vi "Get Pressure.vi"() -> ()   [LabVIEW 2017]
uses:
  Robot Global Data.vi
panel:
  out "Pressure":dbl
  out "Presure Voltage":dbl
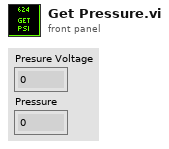
[diagram p1: front panel]
types:
  T1 = typedef "Dashboard Control Data.ctl" = cluster{"Drivetrain Settings Cluster":T2, "Intake Presets":T4, "Elevator Settings Cluster":T5, "Drivetrain Encoder Values":T7, "Auton Chooser":T8, "Auton Presets":cluster{"Start Position":dbl}, "Elevator Encoder Values":T9, "Pressure M":dbl, "Pressure B":dbl}
  T2 = typedef "Drivetrain Settings Cluster.ctl" = cluster{"Gyro Steer PID Gains":T3, "Distance Drive PID Gains":T3, "Drive Tolerance":dbl, "Gyro Tolerance":dbl, "Gyro Output":dbl, "Distance Output":dbl, "Y Power Multiplier":dbl, "Turn Power Multiplier":dbl, "Creep Rate":dbl, "Encoder Reset":bool, "DT Mode Modifier":enum16{"None, Default", "Cube", "Square"}, "Left Encoder Tick Constant":dbl, "Right Encoder Tick Constant":dbl, "Shift Speed":dbl, "Zero Gyro":bool}
  T3 = typedef "PID Gains Cluster.ctl" = cluster{"Integral Time":dbl, "Proportional Gain":dbl, "Derivative Time":dbl}
  T4 = typedef "Intake Presets.ctl" = cluster{"Idle Angle":dbl, "Mid Angle":dbl, "Low Angle":dbl, "Outtake Power":dbl, "Intake Power":dbl, "Unstuck":dbl, "Angle Tolerance":dbl, "Max Angle":dbl, "Max Current":dbl, "Current Trip Time":dbl, "Reset Encoder?":bool, "Encoder Scale":dbl, "PID gains":cluster{"proportional gain (Kc)":dbl, "integral time (Ti, min)":dbl, "derivative time (Td, min)":dbl}, "output range":cluster{"output high":dbl, "output low":dbl}, "IR Constant Pull Rate":dbl}
  T5 = typedef "Elevator Settings Cluster.ctl" = cluster{"Ground Height":dbl, "Switch Height":dbl, "Scale High Height ":dbl, "Scale Low Height":dbl, "Elevator PID Gains":T6, "Elevator Tolerance":dbl, "Reset Encoders":bool, "Encoder Scale":dbl, "Max Height":dbl, "Mid Height":dbl, "output range":cluster{"output high":dbl, "output low":dbl}, "Slow Down Tolerance":dbl, "Tick Constant":dbl, "Anti-tip Multiplier":dbl, "Slow Down Multiplier":dbl}
  T6 = typedef "PID Gains.ctl" = cluster{"proportional gain (Kc)":dbl, "integral time (Ti, min)":dbl, "derivative time (Td, min)":dbl}
  T7 = typedef "DT Encoder Values.ctl" = cluster{"Left Encoder":cluster{"Distance":dbl, "Speed":dbl, "Tick":dbl}, "Right Encoder":cluster{"Distance":dbl, "Speed":dbl, "Tick":dbl}}
  T8 = typedef "Auton Chooser.ctl" = cluster{"Left":bool, "Center":bool, "Right":bool, "Scale":bool, "Both":bool, "Switch":bool}
  T9 = typedef "Elevator Encoder Values.ctl" = cluster{"Encoder Values":cluster{"Distance":dbl, "Speed":dbl, "Tick":dbl}}
  T10 = typedef "WPI_AnalogChannelDevRef.ctl" = cluster{"DevStatus":errorcluster, "Analog Channel":T11}
  T11 = typedef "FPGA_AIChannel.ctl" = enum8{"AI 0", "AI 1", "AI 2", "AI 3", "AI MXP 0", "AI MXP 1", "AI MXP 2", "AI MXP 3", "Invalid"}
  T12 = typedef "Dashboard Status Data.ctl" = cluster{"Elevator Status Cluster":T13, "Drivetrain Status Cluster":T16, "Intake Status Cluster":T18, "Climb Status Cluster":T21, "Intake PDP Info":T22, "Auton Command Cluster":T23, "Pressure ":dbl}
  T13 = typedef "Elevator Status Cluster.ctl" = cluster{"Finished":bool, "Elevator Power":dbl, "Elevator State":T14, "Elevator Mode":T15, "Elevator Height":dbl, "At Bottom?":bool, "At Top?":bool, "Scale high?":bool, "PID Output":dbl}
  T14 = typedef "Elevator State.ctl" = enum16{"Idle", "Ground", "Mid", "Scale", "Switch"}
  T15 = typedef "Elevator Mode.ctl" = enum16{"Semi Auto", "Manual", "Auto"}
  T16 = typedef "Drivetrain Status Cluster.ctl" = cluster{"Throttle (Y)":dbl, "Steer (X)":dbl, "Drivetrain Mode":T17, "Brake?":bool, "Distance Drive Complete?":bool, "PID Drive Complete?":bool, "Creep Mode?":bool, "Gyro Steer Complete?":bool, "Gyro":dbl, "X Max Output":dbl, "X Min Output":dbl, "Y Max Output ":dbl, "Y Min Output":dbl, "Heading Target":dbl, "Distance Target":dbl, "2nd Gear":bool, "Drivetrain Encoder Values":T7}
  T17 = typedef "Drivetrain Mode.ctl" = enum16{"Manual", "Gyro Steer", "PID Drive", "Distance Drive", "Autonomous"}
  T18 = typedef "Intake Status Cluster.ctl" = cluster{"Intake Mode":T19, "Intake States":T20, "Intake Current Angle":dbl, "Cube In Posession?":bool, "Intake Wrist Up?":bool}
  T19 = typedef "Intake Mode.ctl" = enum16{"Auto", "Semi Auto", "Manual"}
  T20 = typedef "Intake States.ctl" = enum16{"Zero", "Override Angle", "Idle", "Drop Mid", "Drop Low", "Outtake", "Intake"}
  T21 = typedef "Climb Status Cluster.ctl" = cluster{"Climb":bool, "Time Remaining":dbl, "Button Pressed":bool}
  T22 = typedef "Intake PDP Info.ctl" = cluster{"Voltage Percent Output":dbl, "Output Voltage":dbl, "Bus Voltage":dbl, "Device ID":dbl, "Output Current":dbl, "Sensor Velocity":dbl, "Sensor Position":dbl, "Pulse Width Position":dbl, "Pulse Width Velocity":dbl, "Temperature":dbl, "Inverted?":bool}
  T23 = typedef "Auton Command Cluster.ctl" = cluster{"commandID":dbl, "headingTarget":dbl, "async":dbl, "elevatorCommand":dbl, "intakeMode":dbl, "maxTime":dbl, "ySpeed":dbl, "zeroGyro":dbl, "intakeCommand":dbl, "distanceTarget":dbl, "xSpeed":dbl, "elevatorMode":dbl, "scaleHigh":dbl, "rollerSpeed":dbl, "intakeAngle":dbl, "manualOpen":dbl, "secondGear":dbl, "elevatorPower":dbl}
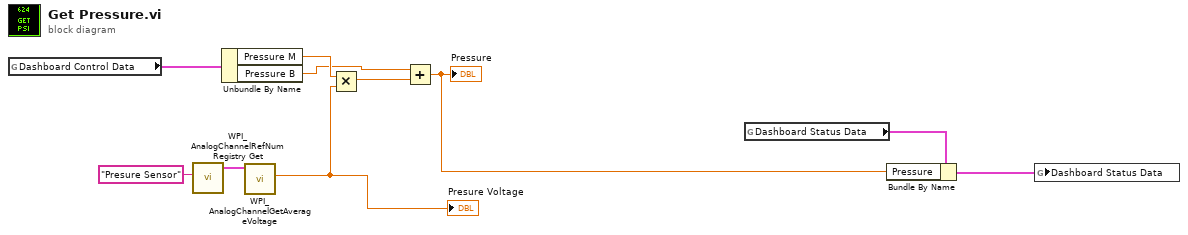
[diagram p0: block diagram]
diagram:
  n1 = global read "Robot Global Data.vi" "Dashboard Control Data"() -> (w8:T1)
  n2 = call <vilib>:"WPI_AnalogChannelRefNum Registry Get.vi"("refnum name"="Presure Sensor") -> ("AIDeviceRef"=w9:T10)  [unwired: 9 in, 1 out]
  n3 = Unbundle By Name(w8) -> ("Pressure M"=w7:dbl, "Pressure B"=w4:dbl)
  n4 = call <vilib>:"WPI_AnalogChannelGetAverageVoltage.vi"("AIDeviceRef"=w9) -> ("Voltage"=w6:dbl)  [unwired: 8 in, 2 out]
  "Presure Voltage" <- w6
  n5 = Multiply(x=w7, y=w6) -> (x*y=w5:dbl)
  n6 = Add(x=w4, y=w5) -> (x+y=w2:dbl)
  "Pressure" <- w2
  n7 = global read "Robot Global Data.vi" "Dashboard Status Data"() -> (w3:T12)
  n8 = Bundle By Name(cluster=w3, "Pressure"=w2) -> (w1:T12)
  n9 = global write "Robot Global Data.vi" "Dashboard Status Data"(w1) -> ()
